vi "Number Of LBCBs 2 Sources.vi"(1 "Number of LBCBs":T2, 2 "Combined LBCBs":bool) -> (0 "Sources":T1[](array[typedef]))   [LabVIEW 2009]
uses:
  Data Access Objects/Application/Number Of LBCBs.ctl
  Dataset Source.ctl
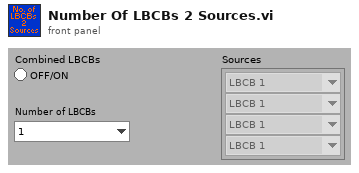
[diagram p1: front panel]
types:
  T1 = typedef "Dataset Source.ctl" = enum16{"LBCB 1", "LBCB 2", "Combined", "External Sensors"}
  T2 = typedef "Number Of LBCBs.ctl" = enum16{"1", "2"}
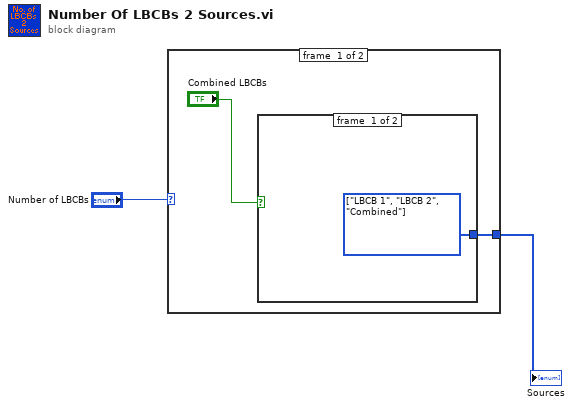
[diagram p0: block diagram]
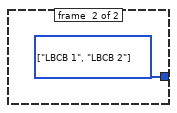
[diagram p2: hidden frame]
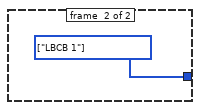
[diagram p3: hidden frame]
diagram:
  n1 = case shown="\"1\"" "Number of LBCBs" {
    tunnel: [w4 w7] -> w1
    frame #0 {
      n2 = case shown="False" "Combined LBCBs" {
        tunnel: [w5 w6] -> w4
        frame #0 {
          w5 = T1[] [enum."LBCB 1", enum."LBCB 2", enum."Combined"] items=["LBCB 1", "LBCB 2", "Combined", "External Sensors"]
        }
        frame #1 {
          w6 = T1[] [enum."LBCB 1", enum."LBCB 2"] items=["LBCB 1", "LBCB 2", "Combined", "External Sensors"]
        }
      }
    }
    frame #1 {
      w7 = T1[] [enum."LBCB 1"] items=["LBCB 1", "LBCB 2", "Combined", "External Sensors"]
    }
  }
  "Sources" <- w1
